vi "Write BLE Message.lvclass.vi"(8 "error in (no error)":errorcluster, 10 "BLE Message.lvclass":refnum<class "BLE Message.lvclass">, 11 "BLE context in":refnum<class "BLE context.lvclass">) -> (0 "error out":errorcluster, 3 "BLE context out":refnum<class "BLE context.lvclass">)   [LabVIEW 2015, in "BLE context.lvclass"]
uses:
  BLE context.lvclass
  BLE Message/BLE Message.lvclass
  BLE context.lvclass/BLE context.ctl
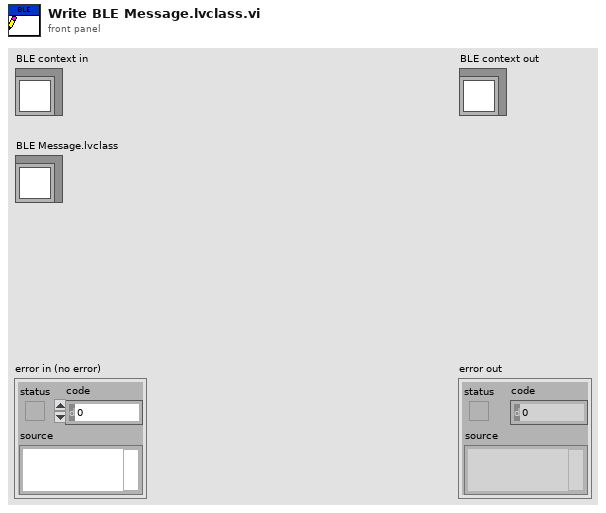
[diagram p1: front panel]
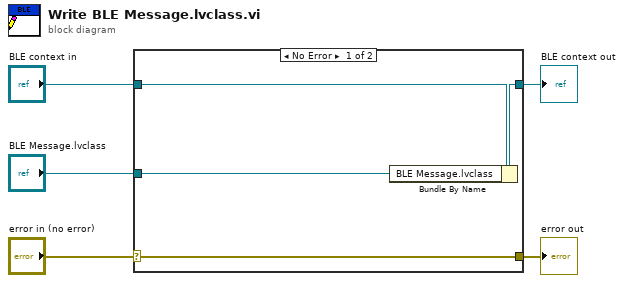
[diagram p0: block diagram]
diagram:
  n1 = case shown="No Error" "error in (no error)" {
    selector: "error in (no error)" -> [w9 w10]
    tunnel: [w9 w10] -> w4
    tunnel: [w7 w11] -> w2
    tunnel: "BLE context in" -> [w8 w11]
    tunnel: "BLE Message.lvclass" -> [w6 _]
    frame No Error {
      n2 = Bundle By Name(cluster=w8, "BLE Message.lvclass"=w6) -> (w7:refnum<class "BLE context.lvclass">)
    }
    frame Error {
    }
  }
  "error out" <- w4
  "BLE context out" <- w2
